vi "controlFixOutputVoltage.vi"(7 "Set":bool, 8 "error in":errorcluster, 9 "Fixed Output Voltage in":dbl, 10 "axis in":u8, 11 "connection ID":refnum<k5>) -> (0 "error out":errorcluster, 1 "Fixed Output Voltage out":dbl, 2 "axis out":u8, 3 "connection ID":refnum<k5>)   [LabVIEW 2016]
panel:
  in  "Set Command":string="com.attocube.amc.control.setControlFixOutputVoltage"
  in  "Get Command":string="com.attocube.amc.control.getControlFixOutputVoltage"
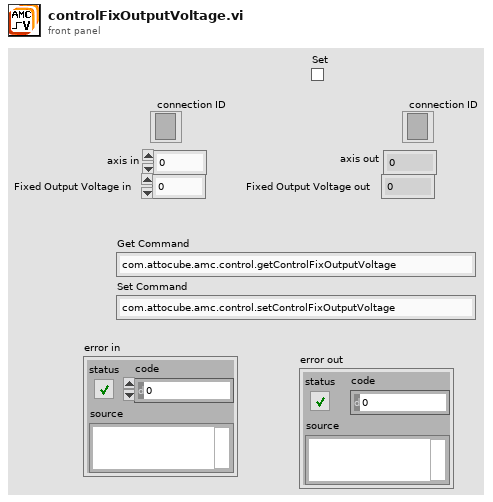
[diagram p1: front panel]
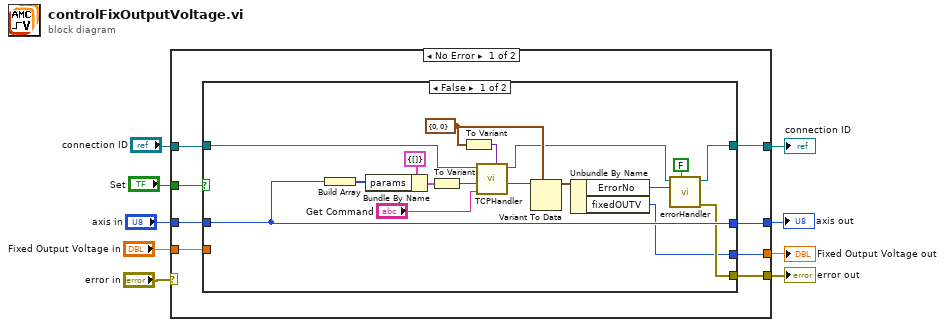
[diagram p0: block diagram]
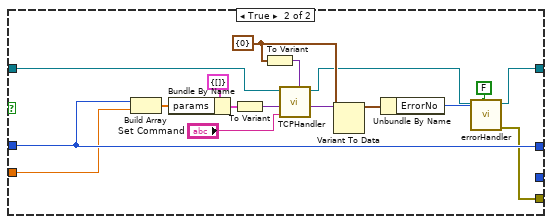
[diagram p2: hidden frame]
diagram:
  n1 = case shown="No Error" "error in" {
    selector: "error in" -> [_ w55]
    tunnel: "axis in" -> [w16 w53]
    tunnel: [w10 w55] -> w8
    tunnel: [w12 w53] -> w7
    tunnel: "Fixed Output Voltage in" -> [w15 w54]
    tunnel: [w11 w54] -> w5
    tunnel: "Set" -> [w17 _]
    tunnel: [w13 w52] -> w3
    tunnel: "connection ID" -> [w14 w52]
    frame No Error {
      n2 = case shown="False" w17 {
        tunnel: [w18 w35] -> w13
        tunnel: w14 -> [w24 w46]
        tunnel: w16 -> [w26 w44]
        tunnel: [w26 w44] -> w12
        tunnel: [w23 _] -> w11
        tunnel: [w25 w41] -> w10
        tunnel: w15 -> [_ w37]
        frame False {
          w21 = cluster{"ErrorNo":i16, "fixedOUTV":i64} {"ErrorNo"=0, "fixedOUTV"=0} ("input cluster")
          n3 = Build Array(w26) -> (w30:u8[])
          n4 = Bundle By Name(cluster=cluster{"params":i16[]} {"params"=[]} ("input cluster"), "params"=w30) -> (w31:cluster{"params":i16[]})
          n5 = To Variant(anything=w31) -> (Variant=w32:variant)
          n6 = To Variant(anything=w21) -> (Variant=w22:variant)
          n7 = call "TCPHandler.vi"("result Types"=w22, "method"="Get Command", "params"=w32, "connection ID"=w24) -> ("result"=w28:variant, "connection ID"=w19:refnum<k5>)  [unwired: 5 in, 1 out]
          n8 = Variant To Data(type=w21, Variant=w28) -> (data=w33:cluster{"ErrorNo":i16, "fixedOUTV":i64})  [unwired: 1 in, 1 out]
          n9 = Unbundle By Name(w33) -> ("ErrorNo"=w34:i16, "fixedOUTV"=w23:i64)
          n10 = call "errorHandler.vi"("show popup"=FALSE, "error number"=w34, "connection ID"=w19) -> ("error out"=w25:errorcluster, "connection ID"=w18:refnum<k5>)  [unwired: 7 in]
        }
        frame True {
          w39 = cluster{"ErrorNo":i16} {"ErrorNo"=0} ("input cluster")
          n11 = Build Array(w44, w37) -> (w48:dbl[])
          n12 = Bundle By Name(cluster=cluster{"params":i64[]} {"params"=[]} ("input cluster"), "params"=w48) -> (w47:cluster{"params":i64[]})
          n13 = To Variant(anything=w47) -> (Variant=w45:variant)
          n14 = To Variant(anything=w39) -> (Variant=w40:variant)
          n15 = call "TCPHandler.vi"("result Types"=w40, "method"="Set Command", "params"=w45, "connection ID"=w46) -> ("result"=w50:variant, "connection ID"=w36:refnum<k5>)  [unwired: 5 in, 1 out]
          n16 = Variant To Data(type=w39, Variant=w50) -> (data=w43:cluster{"ErrorNo":i16})  [unwired: 1 in, 1 out]
          n17 = Unbundle By Name(w43) -> ("ErrorNo"=w42:i16)
          n18 = call "errorHandler.vi"("show popup"=FALSE, "error number"=w42, "connection ID"=w36) -> ("error out"=w41:errorcluster, "connection ID"=w35:refnum<k5>)  [unwired: 7 in]
        }
      }
    }
    frame Error {
    }
  }
  "error out" <- w8
  "axis out" <- w7
  "Fixed Output Voltage out" <- w5
  "connection ID" <- w3
